vi "SetParameter.vi"(8 "error in (no error)":errorcluster, 10 "InClusTiming 2":T1={"Pixelclock"=24, "Exposure"=46.39115, "ExposureTimeBase"=2, "Framerate"=14.99615, "TriggerMode"=0} {"TriggerMode" items=["Auto", "Software", "External sequence start ", "External exposure control"]; "ExposureTimeBase" items=["nanoseconds", "microseconds", "milliseconds"]; "Pixelclock" min=1 max=150 step=1 scale=0.05915..150.0; "Framerate" min=0.05915 max=2000.0 step=1.0 scale=0.05915..100.0 scale format="%#.3g"; "Exposure" min=0.001 max=400.0 step=0.001 scale=0.05915..400.0 scale format="%#.3g"}, 11 "simuCalc in":refnum<class "simuCalc.lvclass">) -> (0 "error out":errorcluster, 3 "simuCalc out":refnum<class "simuCalc.lvclass">)   [LabVIEW 2020, in "simuCalc.lvclass"]
uses:
  simuCalc.lvclass
  simuCalc.lvclass/simuCalc.ctl
  <vilib>/Utility/xml.llb/Read From XML File(string).vi
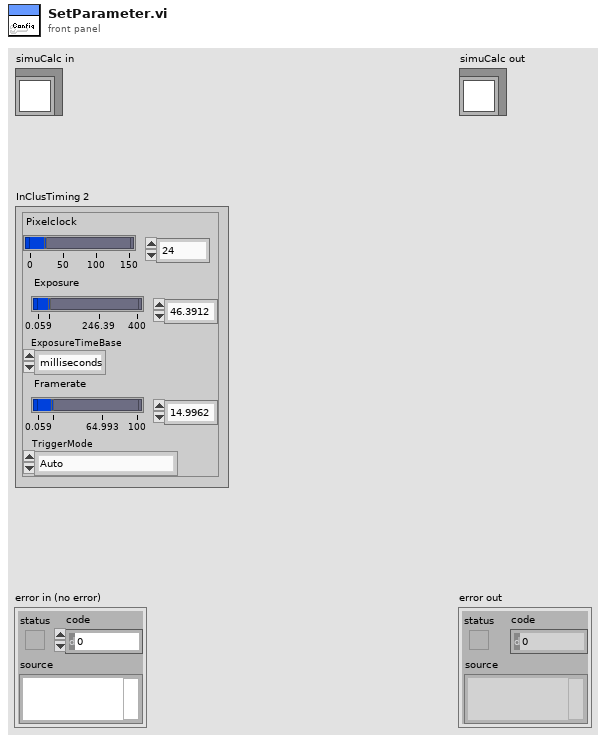
[diagram p1: front panel]
types:
  T1 = cluster{"Pixelclock":i32, "Exposure":dbl, "ExposureTimeBase":u16, "Framerate":dbl, "TriggerMode":u16}
  T2 = cluster{"ROI":cluster{"nbrCol":i32, "nbrlign":i32}, "typeSimu":string}
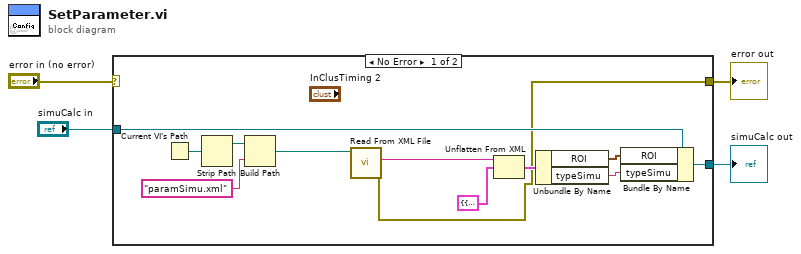
[diagram p0: block diagram]
diagram:
  n1 = case shown="No Error" "error in (no error)" {
    selector: "error in (no error)" -> [_ w18]
    tunnel: [w5 w18] -> w3
    tunnel: "simuCalc in" -> [w7 w17]
    tunnel: [w6 w17] -> w1
    frame No Error {
      n2 = Current VI's Path() -> (path=w9:path)
      n3 = Strip Path(path=w9) -> (stripped path=w8:path)  [unwired: 1 out]
      n4 = Build Path(base path=w8, name or relative path="paramSimu.xml") -> (appended path=w10:path)
      n5 = call-poly <vilib>:"Read From XML File.vi"("XML File Path"=w10) -> ("error out"=w5:errorcluster, "XML Elements"=w16:string)  [unwired: 8 in, 1 out]
      n6 = Unflatten From XML(xml string=w16, type=T2 {"ROI"={"nbrCol"=0, "nbrlign"=0}, "typeSimu"="Random"} ("Cluster of class private data")) -> (value=w14:T2)  [unwired: 1 in, 1 out]
      n7 = Unbundle By Name(w14) -> ("ROI"=w13:cluster{"nbrCol":i32, "nbrlign":i32}, "typeSimu"=w12:string)
      n8 = Bundle By Name(cluster=w7, "ROI"=w13, "typeSimu"=w12) -> (w6:refnum<class "simuCalc.lvclass">)
    }
    frame Error {
    }
  }
  "error out" <- w3
  "simuCalc out" <- w1
